vi "dfd_CH Lowpass S Poles and Zeros.vi"(2 "ripple(dB)":dbl=0.1 format="%.2f", 3 "low cutoff freq: wl":dbl=0.125 format="%.3f", 4 "order":i32=2) -> (0 "zeros":T1[](array[typedef]), 1 "poles":T1[](array[typedef]))   [LabVIEW 2017, in "NI_DigFilter_Design.lvlib"]
uses:
  <vilib>/addons/Digital Filter Design/NI_DigFilter_Design.lvlib
  <vilib>/addons/Digital Filter Design/_Objects.llb/DFD Pole-Zero.ctl
  <vilib>/addons/Digital Filter Design/NI_DigFilterLicensed.lvlib
panel:
  in  "DFD Zero Pole":T1={"value"=0.0+0.0i, "z attr"={"real"=FALSE, "lp"=FALSE, "uc"=FALSE}, "order"=1}
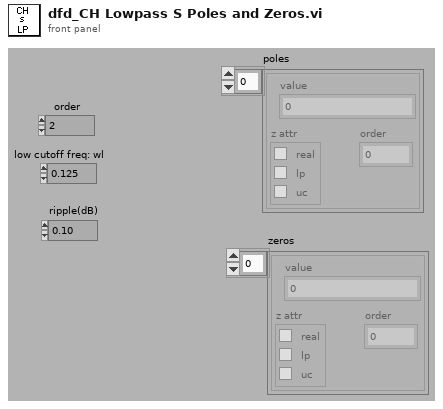
[diagram p1: front panel]
types:
  T1 = typedef "NI_DigFilterLicensed.lvlib/DFD Pole-Zero.ctl" = cluster{"value":cdb, "z attr":cluster{"real":bool, "lp":bool, "uc":bool}, "order":i32}
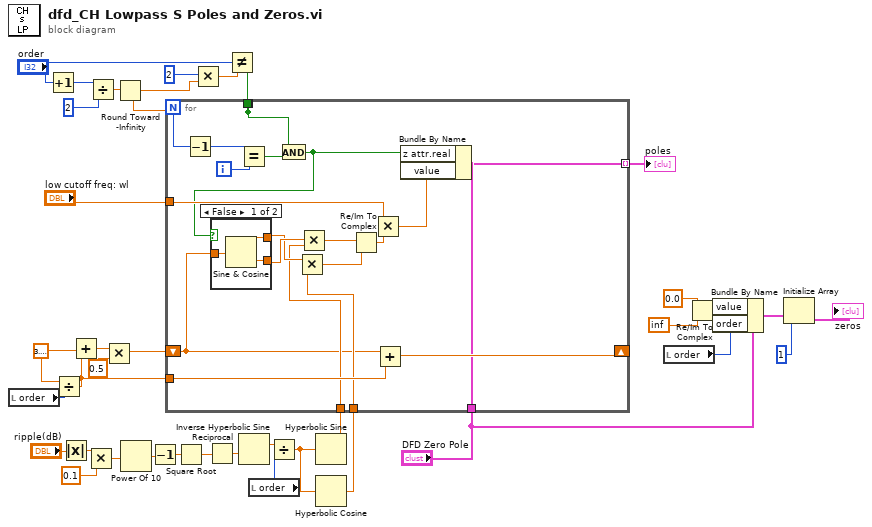
[diagram p0: block diagram]
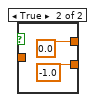
[diagram p2: hidden frame]
diagram:
  w21 = 3.141592653589793
  n1 = local read "order"() -> (w36:i32)
  n2 = Increment(x="order") -> (x+1=w31:i32)
  n3 = Divide(x=w21, y=w36) -> (x/y=w35:dbl)
  n4 = Absolute Value(x="ripple(dB)") -> (abs(x)=w8:dbl)
  n5 = Add(x=w21, y=w35) -> (x+y=w33:dbl)
  n6 = Multiply(x=w8, y=0.1) -> (x*y=w9:dbl)
  n7 = Divide(x=w31, y=2) -> (x/y=w29:dbl)
  n8 = Multiply(x=w33, y=0.5) -> (x*y=w32:dbl)
  n9 = Round Toward -Infinity(1:w29) -> (0:w24:dbl)
  n10 = Power Of 10(x=w9) -> (10^x=w10:dbl)
  n11 = Decrement(x=w10) -> (x-1=w11:dbl)
  n12 = Square Root(x=w11) -> (sqrt(x)=w12:dbl)
  n13 = Multiply(x=2, y=w24) -> (x*y=w26:dbl)
  n14 = Reciprocal(x=w12) -> (1/x=w13:dbl)
  n15 = Not Equal?(x="order", y=w26) -> (x != y?=w25:bool)
  n16 = Inverse Hyperbolic Sine(1:w13) -> (0:w14:dbl)
  n17 = local read "order"() -> (w15:i32)
  n18 = Divide(x=w14, y=w15) -> (x/y=w5:dbl)
  n19 = Hyperbolic Sine(1:w5) -> (0:w4:dbl)
  n20 = Hyperbolic Cosine(1:w5) -> (0:w3:dbl)
  n21 = for {
    N: w24 -> [w52]
    shift-right: [w56] -> _
    shift-left: w32 -> [w39]
    tunnel: w35 -> [w57]
    tunnel: "low cutoff freq: wl" -> [w55]
    tunnel: "DFD Zero Pole" -> [w50]
    tunnel: [w48] -> _ mode=indexing
    tunnel: [w49] -> w28 mode=indexing
    tunnel: w25 -> [w48]
    tunnel: w4 -> [w42]
    tunnel: w3 -> [w41]
    i -> [w54]
    n22 = Decrement(x=w52) -> (x-1=w53:i32)
    n23 = Equal?(x=w53, y=w54) -> (x = y?=w51:bool)
    n24 = And(x=w48, y=w51) -> (x .and. y?=w38:bool)
    n25 = case shown="False" w38 {
      tunnel: w39 -> [w60 _]
      tunnel: [w59 -1.0] -> w45
      tunnel: [w58 0.0] -> w43
      frame False {
        n26 = Sine & Cosine(0:w60) -> (1:w58:dbl, 2:w59:dbl)
      }
      frame True {
      }
    }
    n27 = Multiply(x=w43, y=w41) -> (x*y=w40:dbl)
    n28 = Multiply(x=w45, y=w42) -> (x*y=w44:dbl)
    n29 = Re/Im To Complex(1:w40, 2:w44) -> (0:w47:cdb)
    n30 = Multiply(x=w55, y=w47) -> (x*y=w46:cdb)
    n31 = Add(x=w39, y=w57) -> (x+y=w56:dbl)
    n32 = Bundle By Name(cluster=w50, "z attr.real"=w38, "value"=w46) -> (w49:T1)
  }
  "poles" <- w28
  n33 = local read "order"() -> (w1:i32)
  n34 = Re/Im To Complex(1:inf, 2:0.0) -> (0:w18:cdb)
  n35 = Bundle By Name(cluster="DFD Zero Pole", "value"=w18, "order"=w1) -> (w23:T1)
  n36 = Initialize Array(w23, 1) -> (→"zeros":T1[])
